vi "Run Server.vi"() -> ()   [LabVIEW 2019, in "Service Template.lvlib"]
uses:
  Service Template.lvlib
  <vilib>/gRPC/LabVIEW gRPC Servicer/ServiceBase/ServiceBase.lvclass
  <vilib>/gRPC/LabVIEW gRPC Servicer/Servicer/Servicer.lvclass
panel:
  in  "Async [T] / Sync [F]":bool
  out "Listening Port":i32
  in  "Stop":bool
  in  "Server Address":string="localhost:50051"
  in  "Server Certificate File (.crt)":path
  in  "Server Key File (.key)":path
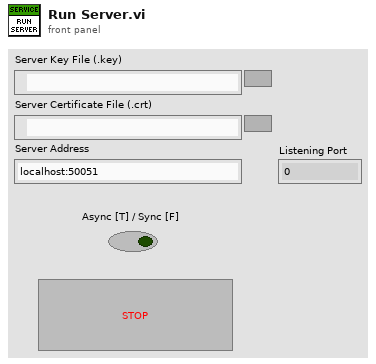
[diagram p1: front panel]
types:
  T1 = enum32{"Invalid", "Standard", "Closed", "Hidden", "Minimized", "Maximized"}
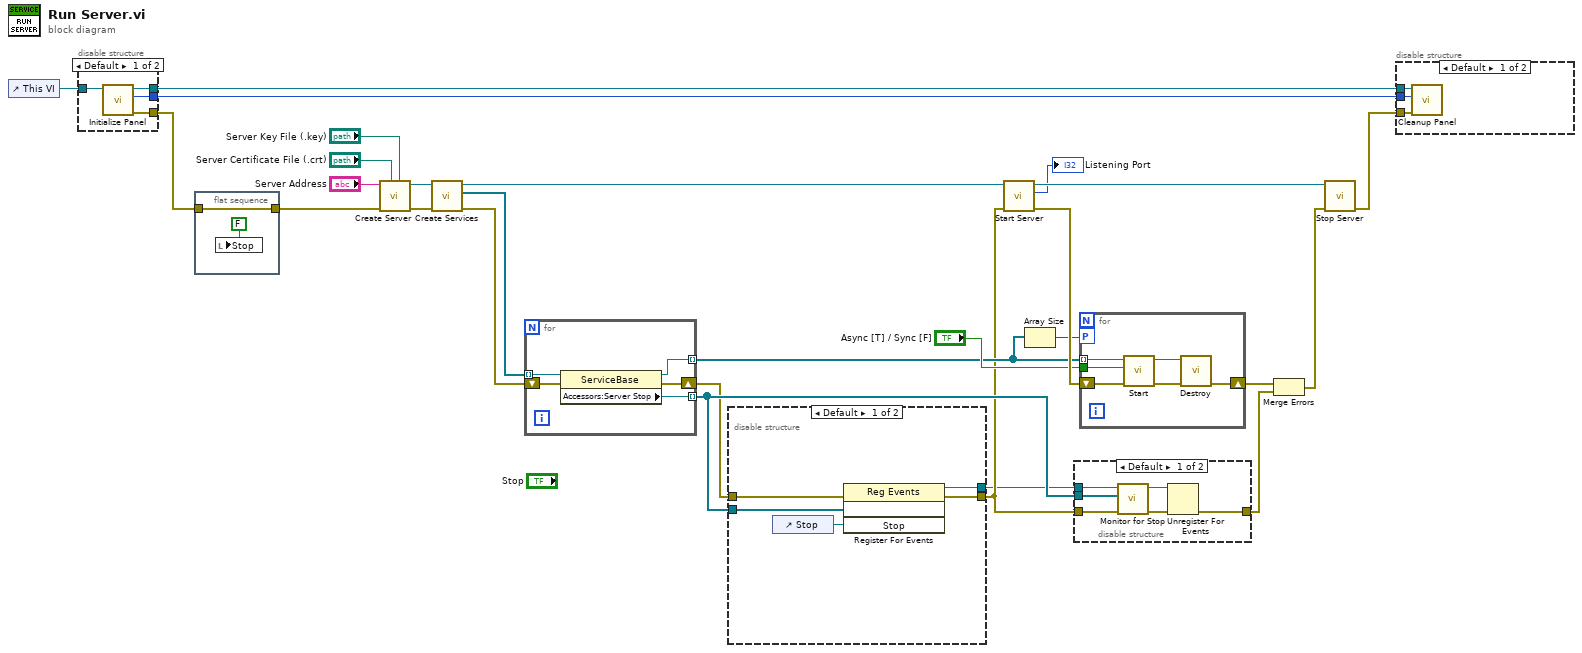
[diagram p0: block diagram]
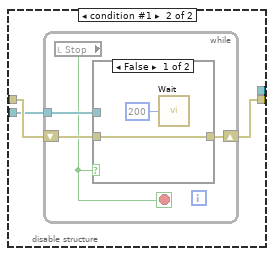
[diagram p2: hidden frame]
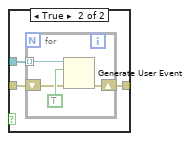
[diagram p3: hidden frame]
diagram:
  n1 = control-ref of="This VI"() -> (w10:refnum<vi>)
  n2 = disable-structure shown="Default" {
    disable-tunnel: [w31 _] -> w2
    disable-tunnel: w10 -> [w30 w32]
    disable-tunnel: [w29 w32] -> w9
    disable-tunnel: [w28 _] -> w8
    frame condition #0 (active) {
      n3 = call "Initialize Panel.vi"("vi reference in"=w30) -> ("error out"=w31:errorcluster, "initial window state"=w28:T1, "vi reference out"=w29:refnum<vi>)  [unwired: 8 in]
    }
    frame condition #1 {
    }
  }
  n4 = flat-sequence {
    tunnel: w2 -> [w34]
    tunnel: [w34] -> w1
    frame #0 {
      n5 = local write "Stop"(FALSE ("Stop")) -> ()
    }
  }
  n6 = call <vilib>:"Create Server.vi"("Server Key File (.key)"="Server Key File (.key)", "Server Certificate File (.crt)"="Server Certificate File (.crt)", "error in"=w1, "Server Address"="Server Address") -> ("error out"=w6:errorcluster, "gRPC server out"=w22:refnum<class "Servicer.lvclass">)  [unwired: 6 in]
  n7 = call "Create Services.vi"("error in (no error)"=w6, "gRPC server in"=w22) -> ("error out"=w5:errorcluster, "gRPC services out"=w4:refnum<class "ServiceBase.lvclass">[], "gRPC server out"=w21:refnum<class "Servicer.lvclass">)  [unwired: 7 in]
  n8 = for {
    tunnel: [w38] -> w16 mode=indexing
    shift-right: [w37] -> w15
    shift-left: w5 -> [w35]
    tunnel: [w39] -> w17 mode=indexing
    tunnel: w4 -> [w36] mode=indexing
    n9 = property class="ServiceBase"(reference=w36, error in=w35) -> (reference out=w39:refnum<class "ServiceBase.lvclass">, error out=w37:errorcluster, "Accessors:Server Stop"=w38:refnum<user-event>)
  }
  n10 = disable-structure shown="Default" {
    disable-tunnel: w16 -> [w44 w46]
    disable-tunnel: w15 -> [w43 w47]
    disable-tunnel: [w42 w45] -> w14
    disable-tunnel: [w40 _] -> w3
    frame condition #0 (active) {
      n11 = control-ref of="Stop"() -> (w41:refnum<vi>)
      n12 = register-events(error in=w43, w44, w41) -> (reference out=w40:refnum<event-registration>, error out=w42:errorcluster)  [unwired: 1 in]
    }
    frame condition #1 {
      n13 = while {
        tunnel: w46 -> [w50]
        shift-right: [w49] -> w45
        shift-left: w47 -> [w51]
        stop <- w48 stop-if-true
        n14 = local read "Stop"() -> (w48:bool)
        n15 = case shown="False" w48 {
          tunnel: [w53 w56] -> w49
          tunnel: w51 -> [w53 w54]
          tunnel: w50 -> [_ w55]
          frame False {
            n16 = call "Wait"("Count(mSec)"=u32 200) -> ()  [unwired: 1 out]
          }
          frame True {
            n17 = for {
              shift-right: [w58] -> w56
              shift-left: w54 -> [w59]
              tunnel: w55 -> [w57] mode=indexing
              n18 = Generate User Event(user event=w57, event data cluster=TRUE ("event data"), error in=w59) -> (error out=w58:errorcluster)  [unwired: 1 in, 1 out]
            }
          }
        }
      }
    }
  }
  n19 = call <vilib>:"Start Server.vi"("error in"=w14, "gRPC server in"=w21) -> ("error out"=w20:errorcluster, "Listening Port"=→"Listening Port":i32, "gRPC server out"=w27:refnum<class "Servicer.lvclass">)  [unwired: 7 in]
  n20 = Array Size(array=w17) -> (size(s)=w18:i32)
  n21 = disable-structure shown="Default" {
    disable-tunnel: w16 -> [w66 _]
    disable-tunnel: w14 -> [w65 w67]
    disable-tunnel: [w63 w67] -> w11
    disable-tunnel: w3 -> [w61 _]
    frame condition #0 (active) {
      n22 = call "Monitor for Stop.vi"("error in (no error)"=w65, "service stop events"=w66, "Event Registration Refnum in"=w61) -> ("error out"=w62:errorcluster, "Event Registration Refnum out"=w64:refnum<event-registration>)  [unwired: 7 in]
      n23 = Unregister For Events(event registration refnum=w64, error in=w62) -> (error out=w63:errorcluster)
    }
    frame condition #1 {
    }
  }
  n24 = for {
    tunnel: w17 -> [w71] mode=indexing
    tunnel: "Async [T] / Sync [F]" -> [w69]
    workers-P: w18 -> [_]
    shift-right: [w68] -> w13
    shift-left: w20 -> [w70]
    n25 = call-dynamic "Start.vi"("error in"=w70, "ASync [T]"=w69, "gRPC service in"=w71) -> ("error out"=w72:errorcluster, "gRPC service out"=w73:refnum<class "ServiceBase.lvclass">)  [unwired: 7 in]
    n26 = call-dynamic "Destroy.vi"("error in"=w72, "gRPC service in"=w73) -> ("error out"=w68:errorcluster)  [unwired: 8 in, 1 out]
  }
  n27 = Merge Errors(w13, w11) -> (w12:errorcluster)
  n28 = call <vilib>:"Stop Server.vi"("error in"=w12, "gRPC server in"=w27) -> ("error out"=w7:errorcluster)  [unwired: 9 in]
  n29 = disable-structure shown="Default" {
    disable-tunnel: w9 -> [w76 _]
    disable-tunnel: w8 -> [w75 _]
    disable-tunnel: w7 -> [w74 _]
    frame condition #0 (active) {
      n30 = call "Cleanup Panel.vi"("error in (no error)"=w74, "initial window state"=w75, "vi reference in"=w76) -> ()  [unwired: 7 in, 2 out]
    }
    frame condition #1 {
    }
  }
